vi "AMP_Modbus_TCP.vi"() -> ()   [LabVIEW 2014]
uses:
  <vilib>/Plasmionique/MB Master/MB_Master_TCP/MB_Master_TCP.lvclass
  <vilib>/Plasmionique/MB Master/MB Master.lvlib
panel:
  out "Actual Velocity  rps  40011":i32
  out "Encoder Position 40005..40006":i32
  out "Read first 50 Holding Registers":dbl[](array[numeric])
  in  "Stop":bool
  in  "WriteData":bool
  in  "Deceleration rps/s":u16
  in  "Acceleration rps/s":u16
  in  "Velocity rps":u16
  out "Decimal value":i16
  in  "Write Opcode Value to register  40125 values in Hex as per manual":string
  in  "Point to Point Distance":i32
  in  "Remote Port":u16=502
  in  "Remote IP Address":string="192.168.1.15"
  out "error out":errorcluster
  in  "error in":errorcluster
  # "Applied Motion Products Modbus TCP example\n\nInstructions\n1.Use product manual to set IP address of the device and enter in \n\"Remote IP Addres\"\n2. Run this VI\n3. Change value of parameters and  press \"Write Data\""
  # "Read Holding Registers"
  # "Write Holding Registers"
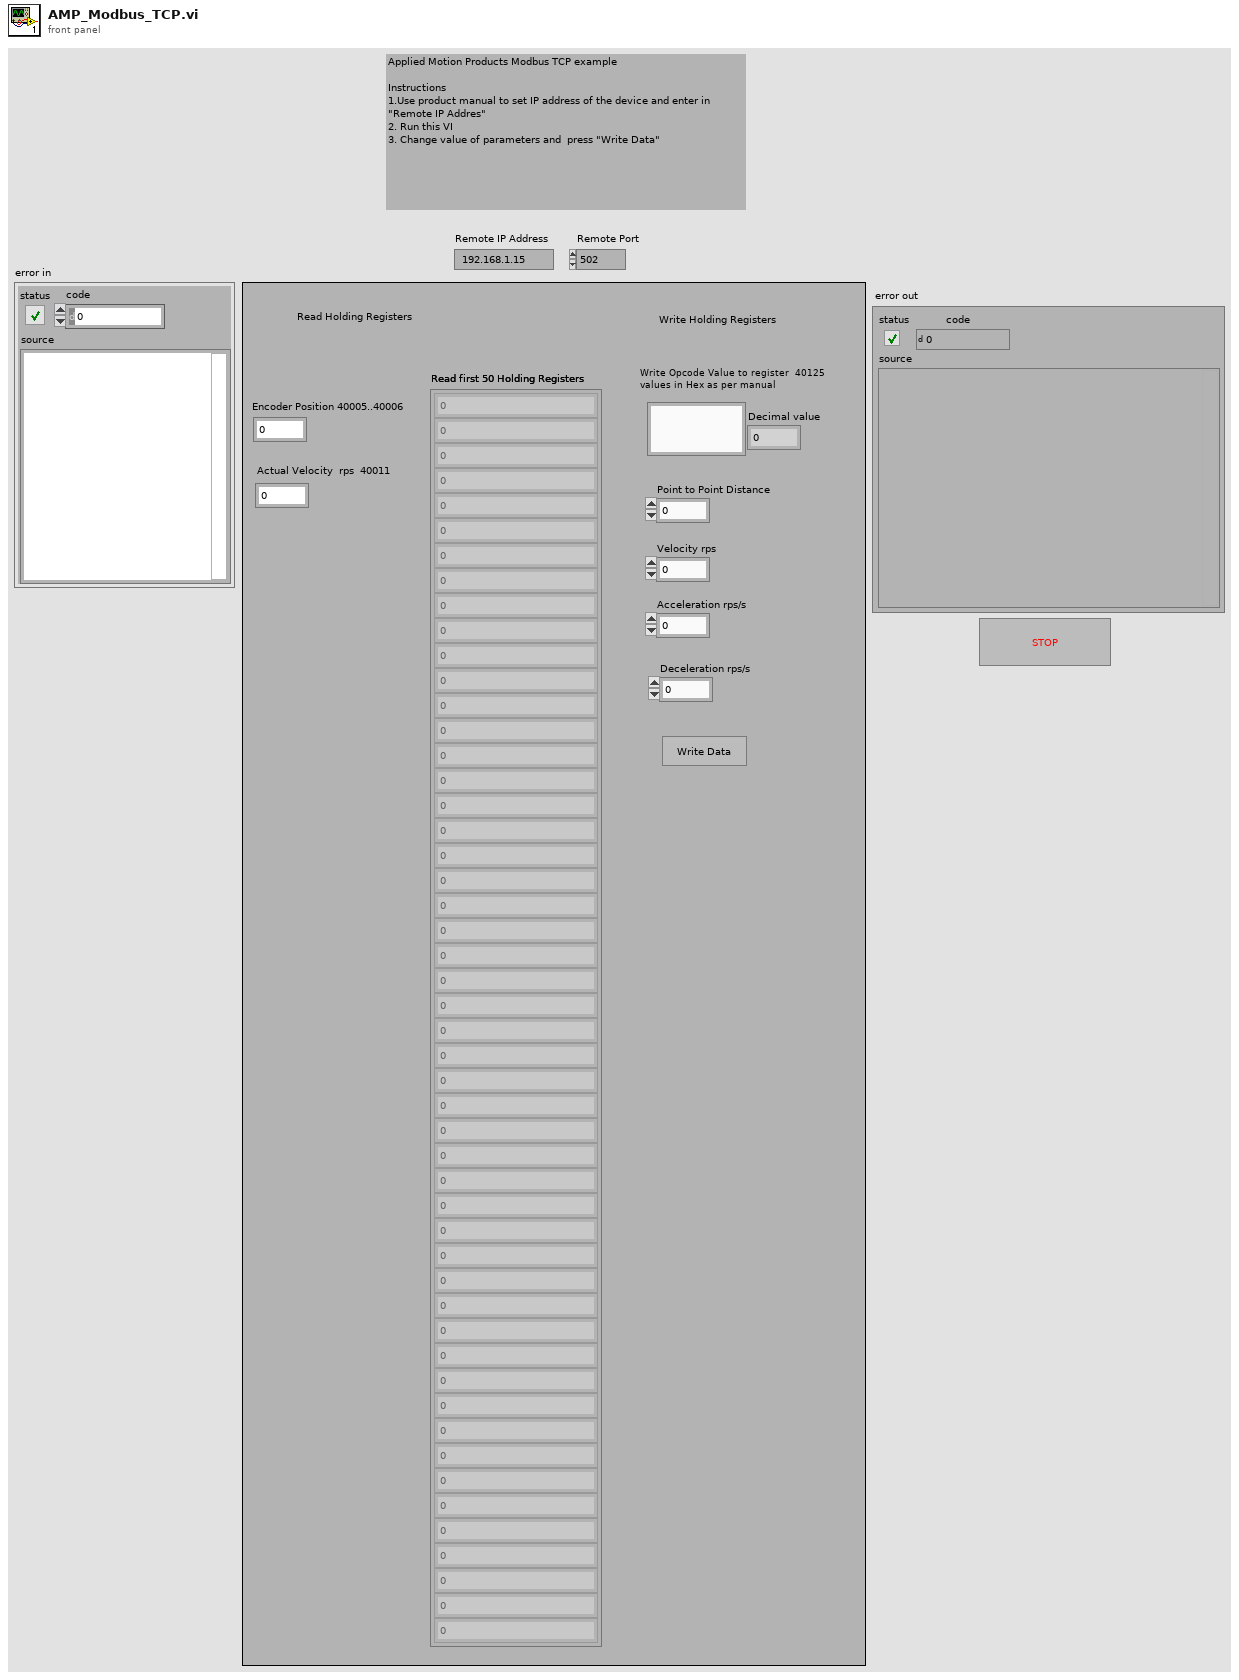
[diagram p1: front panel]
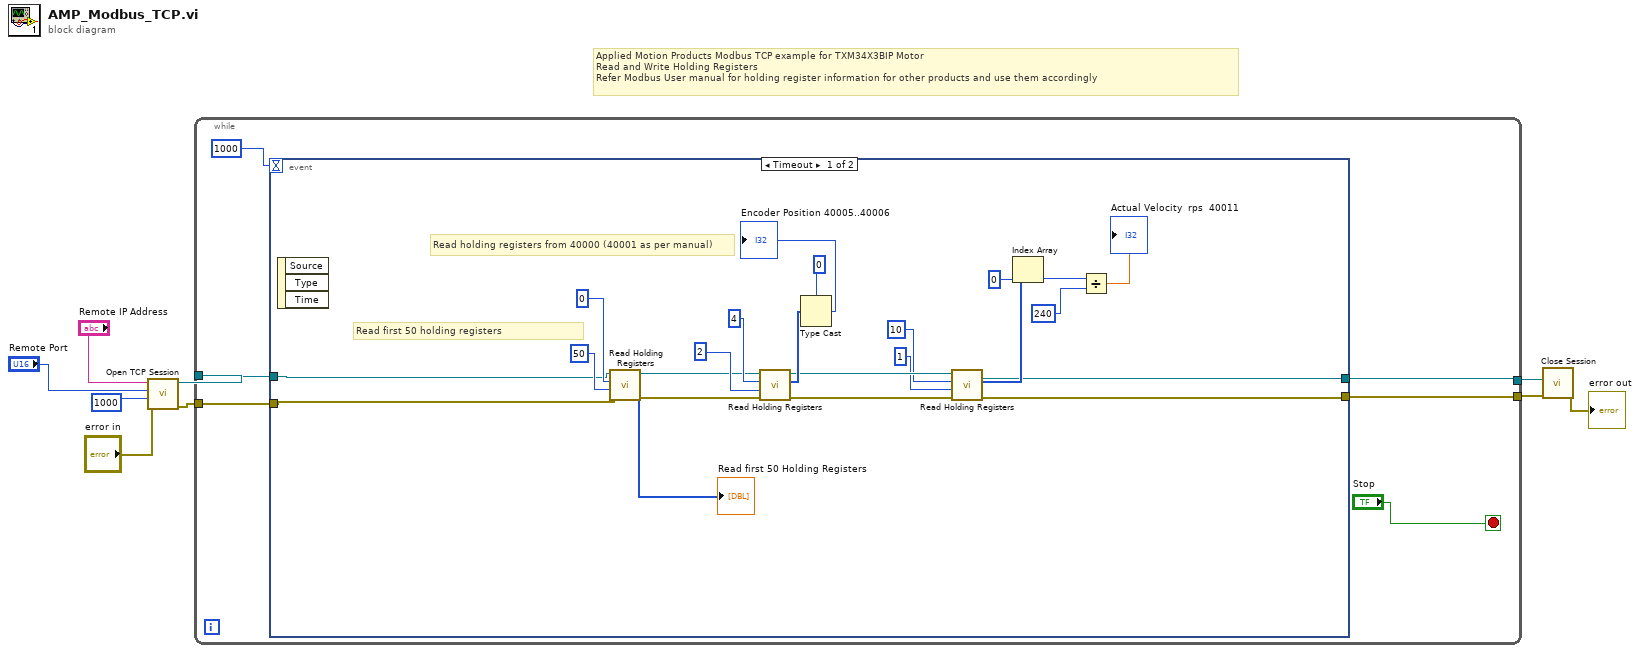
[diagram p0: block diagram]
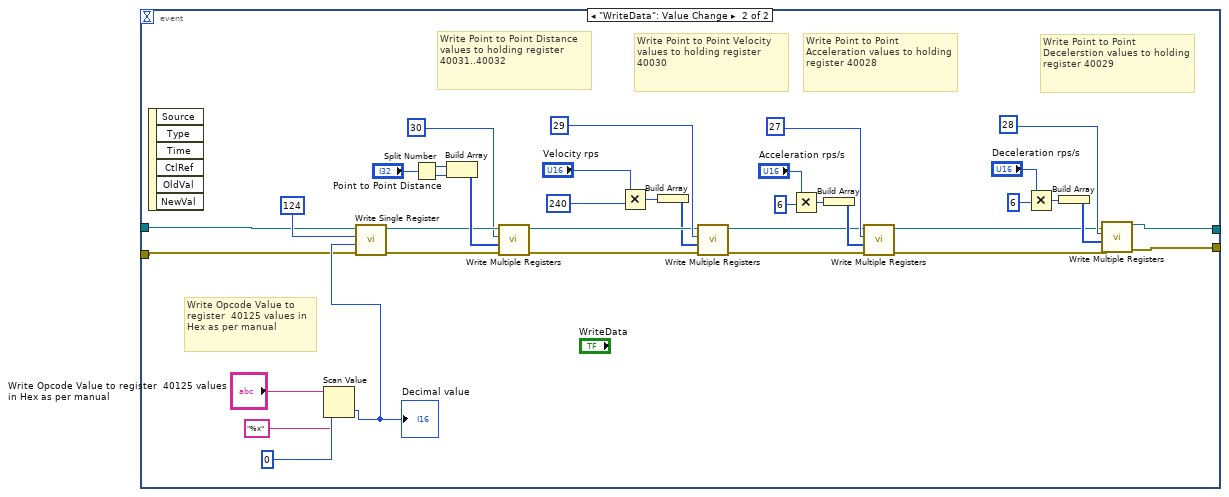
[diagram p2: hidden frame]
diagram:
  # "Applied Motion Products Modbus TCP example for TXM34X3BIP Motor\nRead and Write Holding Registers\nRefer Modbus User manual for holding register information for other products and use them accordingly"
  n1 = call <vilib>:"Open TCP Session.vi"("error in (no error)"="error in", "Timeout (10000)"=1000 ("connect timeout ms"), "Port (502)"="Remote Port", "IP Address"="Remote IP Address") -> ("error out"=w7:errorcluster, "MB_TCP session"=w6:refnum<class "MB_Master_TCP.lvclass">)  [unwired: 6 in]
  n2 = while {
    tunnel: w6 -> [w15]
    tunnel: w7 -> [w14]
    tunnel: [w13] -> w5
    tunnel: [w11] -> w3
    stop <- "Stop" stop-if-true
    n3 = event shown="[0] Timeout" {
      selector: _ -> [_ _]
      dyn-events: _ -> [_ _]
      timeout: u32 1000 ("milliseconds to wait") -> [_ _]
      tunnel: w15 -> [w19 w39]
      tunnel: w14 -> [w18 w40]
      tunnel: [w17 w42] -> w13
      tunnel: [w16 w41] -> w11
      event Timeout {
        # "Read first 50 holding registers"
        # "Read holding registers from 40000 (40001 as per manual)"
        n4 = event-data() -> ()  [unwired: 1 in, 3 out]
        n5 = call <vilib>:"Read Holding Registers.vi"("error in (no error)"=w18, "quantity"=50, "starting address"=0, "MB session in"=w19) -> ("error out"=w33:errorcluster, "Registers"=→"Read first 50 Holding Registers":u16[], "MB session out"=w32:refnum<class "MB_Master_TCP.lvclass">)  [unwired: 5 in]
        n6 = call <vilib>:"Read Holding Registers.vi"("error in (no error)"=w33, "quantity"=2, "starting address"=4, "MB session in"=w32) -> ("error out"=w30:errorcluster, "Registers"=w35:u16[], "MB session out"=w31:refnum<class "MB_Master_TCP.lvclass">)  [unwired: 5 in]
        n7 = Type Cast(type=0, x=w35) -> (*(type *) &x=→"Encoder Position 40005..40006":i32)
        n8 = call <vilib>:"Read Holding Registers.vi"("error in (no error)"=w30, "quantity"=1, "starting address"=10, "MB session in"=w31) -> ("error out"=w16:errorcluster, "Registers"=w21:u16[], "MB session out"=w17:refnum<class "MB_Master_TCP.lvclass">)  [unwired: 5 in]
        n9 = Index Array(array=w21, index=0) -> (element=w23:u16)
        n10 = Divide(x=w23, y=240) -> (x/y=→"Actual Velocity  rps  40011":dbl)
      }
      event "WriteData": Value Change {
        # "Write Point to Point Decelerstion values to holding register 40029"
        # "Write Point to Point Acceleration values to holding register 40028"
        # "Write Opcode Value to register  40125 values in Hex as per manual"
        # "Write Point to Point Velocity values to holding register 40030"
        # "Write Point to Point Distance values to holding register 40031..40032"
        n11 = event-data() -> ()  [unwired: 1 in, 6 out]
        n12 = Scan Value(string="Write Opcode Value to register  40125 values in Hex as per manual", format string="%x", default (0 dbl)=0) -> (value=w64:i32)  [unwired: 1 out]
        "Decimal value" <- w64
        n13 = call <vilib>:"Write Single Register.vi"("error in (no error)"=w40, "value"=w64, "address"=u16 124 ("Write Opcode command\nHolding Register 40125"), "MB session in"=w39) -> ("error out"=w70:errorcluster, "MB session out"=w71:refnum<class "MB_Master_TCP.lvclass">)  [unwired: 6 in]
        n14 = Split Number(x="Point to Point Distance") -> (hi(x)=w74:u16, lo(x)=w73:u16)
        n15 = Build Array(w74, w73) -> (w72:u16[])
        n16 = call <vilib>:"Write Multiple Registers.vi"("error in (no error)"=w70, "values"=w72, "starting address"=u16 30 ("Write Opcode command\nHolding Register 40125"), "MB session in"=w71) -> ("error out"=w62:errorcluster, "MB session out"=w61:refnum<class "MB_Master_TCP.lvclass">)  [unwired: 6 in]
        n17 = Multiply(x="Velocity rps", y=u16 240 ("Write Opcode command\nHolding Register 40125")) -> (x*y=w57:u16)
        n18 = Build Array(w57) -> (w60:u16[])
        n19 = call <vilib>:"Write Multiple Registers.vi"("error in (no error)"=w62, "values"=w60, "starting address"=u16 29 ("Write Opcode command\nHolding Register 40125"), "MB session in"=w61) -> ("error out"=w44:errorcluster, "MB session out"=w46:refnum<class "MB_Master_TCP.lvclass">)  [unwired: 6 in]
        n20 = Multiply(x="Acceleration rps/s", y=u16 6 ("Write Opcode command\nHolding Register 40125")) -> (x*y=w52:u16)
        n21 = Build Array(w52) -> (w55:u16[])
        n22 = call <vilib>:"Write Multiple Registers.vi"("error in (no error)"=w44, "values"=w55, "starting address"=u16 27 ("Write Opcode command\nHolding Register 40125"), "MB session in"=w46) -> ("error out"=w43:errorcluster, "MB session out"=w45:refnum<class "MB_Master_TCP.lvclass">)  [unwired: 6 in]
        n23 = Multiply(x="Deceleration rps/s", y=u16 6 ("Write Opcode command\nHolding Register 40125")) -> (x*y=w47:u16)
        n24 = Build Array(w47) -> (w50:u16[])
        n25 = call <vilib>:"Write Multiple Registers.vi"("error in (no error)"=w43, "values"=w50, "starting address"=u16 28 ("Write Opcode command\nHolding Register 40125"), "MB session in"=w45) -> ("error out"=w41:errorcluster, "MB session out"=w42:refnum<class "MB_Master_TCP.lvclass">)  [unwired: 6 in]
      }
    }
  }
  n26 = call-dynamic "Close Session.vi"("error in (no error)"=w3, "MB TCP session"=w5) -> ("error out"=→"error out":errorcluster)  [unwired: 9 in]
